vi "Arm Command.vi"(7 "Description":string, 8 "Command Info In":T2, 11 "SubSystem Data":T1) -> (0 "Command Info Out":T2)   [LabVIEW 2023]
doc: "This template is useful for immediate subsystem actions that do not need deadband filtering\n\nBe sure to right-click and select New from Template and save with a new command name."
uses:
  <vilib>/Rock Robotics/WPI/Framework/Command Status Info.ctl
  <vilib>/Rock Robotics/WPI/Framework/Completion Status.ctl
  <vilib>/Rock Robotics/WPI/Framework/Completion Notifier.ctl
  Implementation/Arm Setpoints.ctl
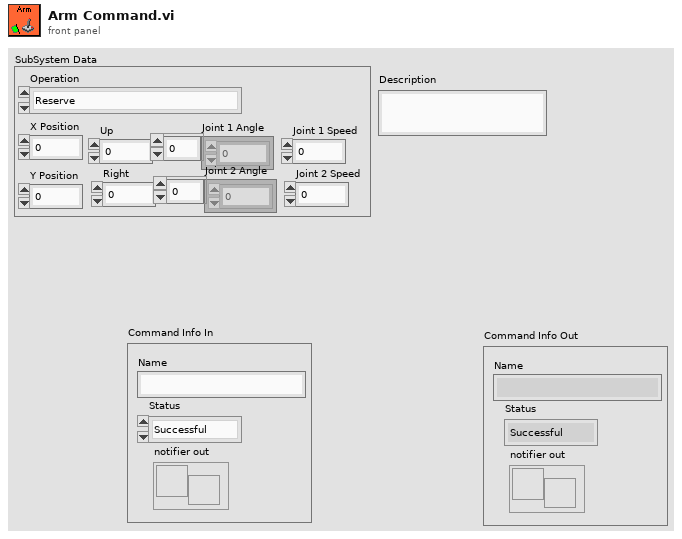
[diagram p1: front panel]
types:
  T1 = typedef "Arm Setpoints.ctl" = cluster{"Operation":enum16{"Reserve", "Read Current", "Immediate", "Move to position", "Adjust position", "Cube extend", "Cone extend", "Rotate Arm Joints", "Maintain Angle", "Retract", "Go_to_next"}, "X Position":dbl, "Y Position":dbl, "Up":dbl, "Right":dbl, "Joint 1 Angle":dbl[], "Joint 2 Angle":dbl[], "Joint 1 Speed":dbl, "Joint 2 Speed":dbl}
  T2 = typedef "Command Status Info.ctl" = cluster{"Name":string, "Status":T3, "notifier out":T4}
  T3 = typedef "Completion Status.ctl" = enum16{"Successful", "Aborted", "Incomplete"}
  T4 = typedef "Completion Notifier.ctl" = refnum<notifier>
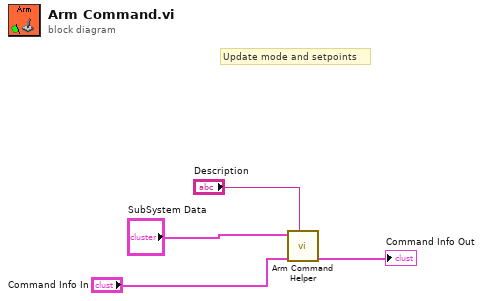
[diagram p0: block diagram]
diagram:
  # "Update mode and setpoints"
  n1 = call "Arm Command Helper.vi"("Description"="Description", "Command Info In"="Command Info In", "SubSystem Data"="SubSystem Data") -> ("Command Info Out"=→"Command Info Out":T2)  [unwired: 6 in, 2 out]
